vi "init.vi"(8 "error in (no error)":errorcluster, 11 "DualActingPneumaticCylinder_Axial in":refnum<class "DualActingPneumaticCylinder_Axial.lvclass">) -> (0 "error out":errorcluster, 3 "DualActingPneumaticCylinder_Axial out":refnum<class "DualActingPneumaticCylinder_Axial.lvclass">)   [LabVIEW 2013, in "DualActingPneumaticCylinder_Axial.lvclass"]
uses:
  DualActingPneumaticCylinder_Axial.lvclass
  PressureTransducerCompensator_Axial/PressureTransducerCompensator_Axial.lvclass
  FlowControlValveCompensator_Axial/FlowControlValveCompensator_Axial.lvclass
  DualActingPneumaticCylinder/DualActingPneumaticCylinder.lvclass/DualActingPneumaticCylinder.ctl
  PressureTransducerCompensator/PressureTransducerCompensator.lvclass
  FlowControlValveCompensator/FlowControlValveCompensator.lvclass
  DualActingPneumaticCylinder/DualActingPneumaticCylinder.lvclass
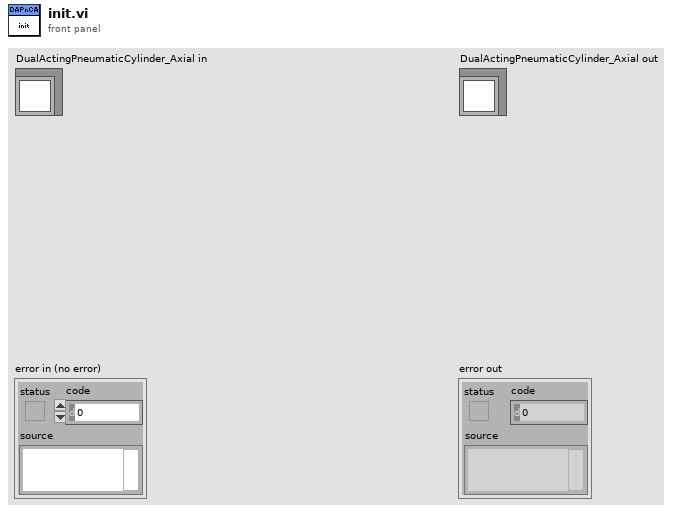
[diagram p1: front panel]
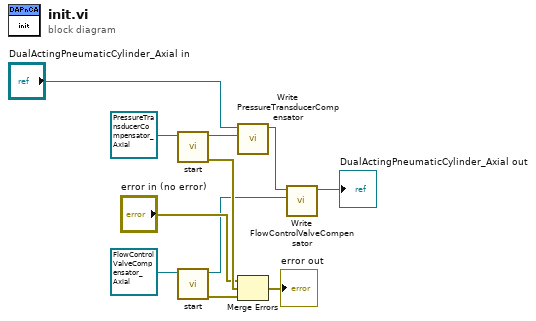
[diagram p0: block diagram]
diagram:
  n1 = call "start.vi"("PressureTransducerCompensator in"=refnum<class "PressureTransducerCompensator_Axial.lvclass"> refnum ("PressureTransducerCompensator_Axial.lvclass")) -> ("error out"=w9:errorcluster, "PressureTransducerCompensator out"=w11:refnum<class "PressureTransducerCompensator_Axial.lvclass">)  [unwired: 9 in]
  n2 = call "start.vi"("FlowControlValveCompensator in"=refnum<class "FlowControlValveCompensator_Axial.lvclass"> refnum ("FlowControlValveCompensator_Axial.lvclass")) -> ("error out"=w10:errorcluster, "FlowControlValveCompensator out"=w3:refnum<class "FlowControlValveCompensator_Axial.lvclass">)  [unwired: 9 in]
  n3 = call "Write PressureTransducerCompensator.vi"("PressureTransducerCompensator.lvclass"=w11, "DualActingPneumaticCylinder in"="DualActingPneumaticCylinder_Axial in") -> ("DualActingPneumaticCylinder out"=w4:refnum<class "DualActingPneumaticCylinder_Axial.lvclass">)  [unwired: 9 in]
  n4 = Merge Errors("error in (no error)", w9, w10) -> (→"error out":errorcluster)
  n5 = call "Write FlowControlValveCompensator.vi"("FlowControlValveCompensator.lvclass"=w3, "DualActingPneumaticCylinder in"=w4) -> ("DualActingPneumaticCylinder out"=→"DualActingPneumaticCylinder_Axial out":refnum<class "DualActingPneumaticCylinder_Axial.lvclass">)  [unwired: 9 in]
